vi "Detect Edge.vi"(10 "Edge Type?":enum16{"Rising", "Falling"}(ring), 11 "Signal In":bool) -> (3 "Edge Detected?":bool)   [LabVIEW 2015]
doc: "This VI takes in a digital signal one point at a time and detects either a rising edge or a falling edge based on the input option specified."
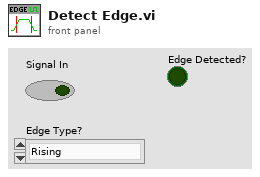
[diagram p1: front panel]
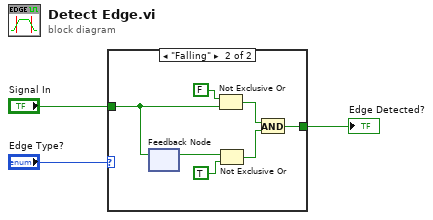
[diagram p0: block diagram]
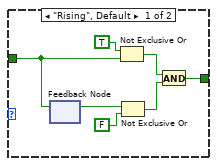
[diagram p2: hidden frame]
diagram:
  n1 = case shown="\"Falling\"" "Edge Type?" {
    tunnel: "Signal In" -> [w10 w17]
    tunnel: [w4 w11] -> w1
    frame "Rising", Default {
      n2 = feedback-in #1(w10) -> ()
      n3 = feedback #1() -> (w9:bool)  [unwired: 1 in]
      n4 = Not Exclusive Or(1:w10, 2:TRUE ("x")) -> (0:w5:bool)
      n5 = Not Exclusive Or(1:FALSE ("y"), 2:w9) -> (0:w6:bool)
      n6 = And(x=w5, y=w6) -> (x .and. y?=w4:bool)
    }
    frame "Falling" {
      n7 = feedback-in #2(w17) -> ()
      n8 = feedback #2() -> (w16:bool)  [unwired: 1 in]
      n9 = Not Exclusive Or(1:w17, 2:FALSE ("x")) -> (0:w12:bool)
      n10 = Not Exclusive Or(1:TRUE ("y"), 2:w16) -> (0:w13:bool)
      n11 = And(x=w12, y=w13) -> (x .and. y?=w11:bool)
    }
  }
  "Edge Detected?" <- w1
